vi "NI XNET CAN Signal and DAQ Logger.vi"() -> ()   [LabVIEW 2021, in "XNET-CAN-Signal-Logger.lvlib"]
uses:
  XNET-CAN-Signal-Logger.lvlib
  Typedef/Def-CAN Port Configuration.ctl
  Typedef/Def-Signal to Monitor.ctl
  Typedef/Def-DAQ AI Configuration.ctl
  Typedef/Def-Logging State.ctl
  Typedef/Def-Data Queue Ref.ctl
  Typedef/Def-Data Queue Type.ctl
  <userlib>/_NEVSTOP/NEVSTOP_TimerEngine/_Typedef/Timer-UserEvent.ctl
  Typedef/Def-GSTOP.ctl
  SubVIs/Global Variables.vi
  <userlib>/_NEVSTOP/GlobalStop/_gStop.vi
  <resource>/objmgr/xnet.rc
  <userlib>/_NEVSTOP/GlobalStop/GSTOP.lvlib
  <userlib>/_NEVSTOP/NEVSTOP_TimerEngine/TimerEngine.lvclass
panel:
  out "File size":i64 caption="File size:" format="%.0f MB"
  out "State":string caption="State:"
  in  "Tab Control":enum32{"CAN", "Analog Input"}(tab)
  in  "CAN Configurations":T1[](array[typedef]) {"Sample Rate (Hz)" format="%#_13g"}
  in  "DAQ AI Configurations":T2[](array[typedef]) {"Terminal Config" items=["Default"=-1, "RSE"=10083, "NRSE"=10078, "Differential"=10106, "Pseudodifferential"=12529]; "Min (V)" format="%#_13g"; "Max (V)" format="%#_13g"; "Sample Rate (Hz)" format="%#_13g"}
  in  "Stop Logging":bool
  in  "Signal to Monitor":T3[](array[typedef])
  out "# elements in queue":i32 caption="# elements in queue:"
  in  "Start Logging":bool
  out "Preview":string caption="Preview:"
  in  "Log file name":string="LogFile_{Year}-{Month}-{Day}-{Hour}-{Minute}-{Second}.tdms"
  in  "Log file folder":path=path "C:/Users/NI/Desktop/Data"
  in  "Exit":bool
  in  "Segment Files":bool=TRUE
  in  "Segment File Size":i64=100 caption="Seg File Size" format="%.0f MB"
  # "Configuration"
  # "Signals to Monitor"
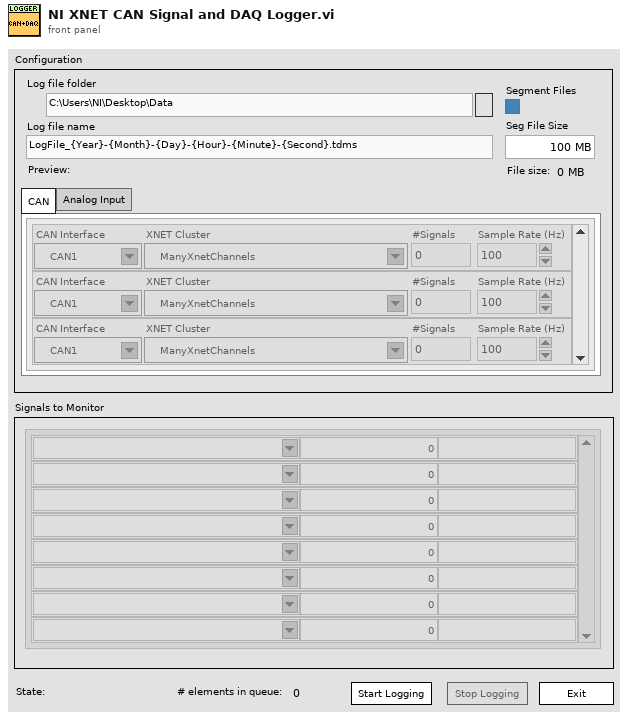
[diagram p1: front panel]
types:
  T1 = typedef "XNET-CAN-Signal-Logger.lvlib/Def-CAN Port Configuration.ctl" = cluster{"CAN Interface":refnum<k21>, "XNET Cluster":refnum<k21>, "#Signals":i32, "Sample Rate (Hz)":dbl}
  T2 = typedef "XNET-CAN-Signal-Logger.lvlib/Def-DAQ AI Configuration.ctl" = cluster{"AI Channels":tag, "Min (V)":dbl, "Max (V)":dbl, "Terminal Config":i32, "Sample Rate (Hz)":dbl, "#Samples":i32}
  T3 = typedef "XNET-CAN-Signal-Logger.lvlib/Def-Signal to Monitor.ctl" = cluster{"Name":string, "Value":dbl, "Unit":string}
  T4 = enum32{"Invalid", "Standard", "Closed", "Hidden", "Minimized", "Maximized"}
  T5 = enum32{"invalid app kind", "Development System", "Run Time System", "Student Edition", "Embedded LabVIEW", "Evaluation", "Custom"}
  T6 = enum8{"Enabled", "Disabled", "Disabled and Grayed Out"}
  T7 = typedef "XNET-CAN-Signal-Logger.lvlib/Def-Logging State.ctl" = enum16{"Configuring", "Logging..."}
  T8 = typedef "XNET-CAN-Signal-Logger.lvlib/Def-Data Queue Type.ctl" = cluster{"PackageID":i32, "Data":waveform(dbl)[]}
  T9 = typedef "XNET-CAN-Signal-Logger.lvlib/Def-GSTOP.ctl" = enum16{"Writer", "Readers"}
  T10 = typedef "XNET-CAN-Signal-Logger.lvlib/Def-Data Queue Ref.ctl" = refnum<queue>
  T11 = cluster{"Core":cluster{"Current VI Reference":refnum<vi>, "Close Panel on Exit?":bool}, "Logging State":T7, "LogFilePath":path, "Data Queue Ref":T10, "Error Queue Ref":refnum<queue>, "Monitor.SignalNames":string[], "Monitor.SignalUnits":string[]}
  T12 = cluster{"Current VI Reference":refnum<vi>, "Close Panel on Exit?":bool}
  T13 = typedef "TimerEngine.lvlib/TimerEngine.lvclass/Timer-UserEvent.ctl" = refnum<user-event>
  T14 = typedef "TimerEngine.lvlib/TimerEngine.lvclass/Timer-Userevent.ctl" = refnum<user-event>
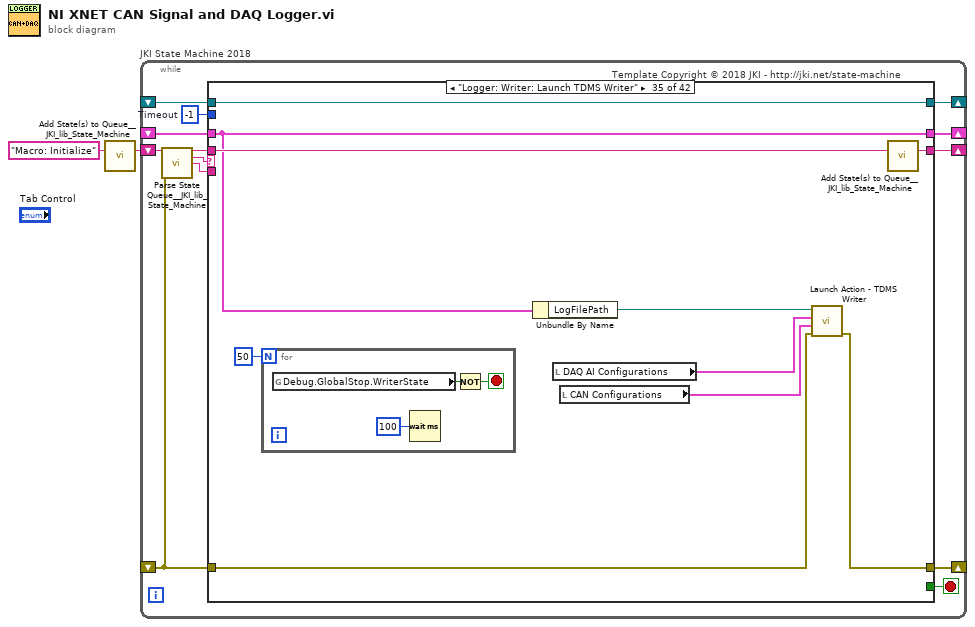
[diagram p0: block diagram]
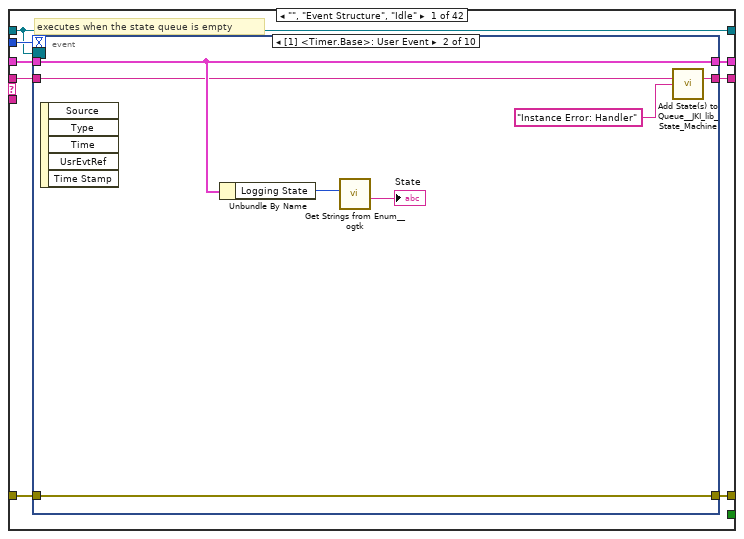
[diagram p2: hidden frame]
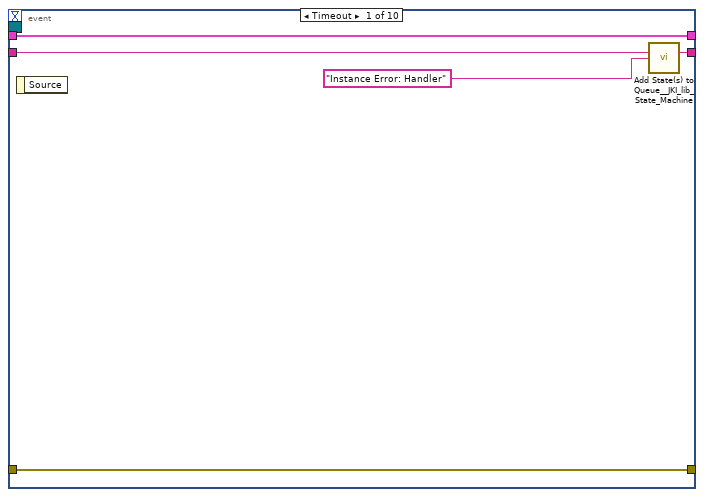
[diagram p3: hidden frame]
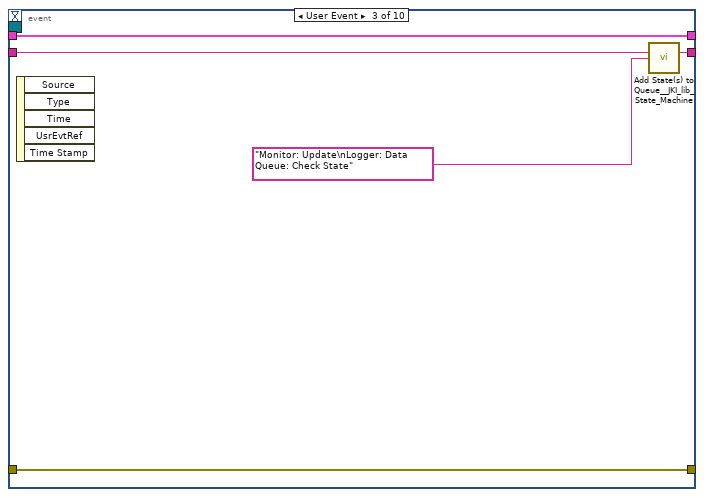
[diagram p4: hidden frame]
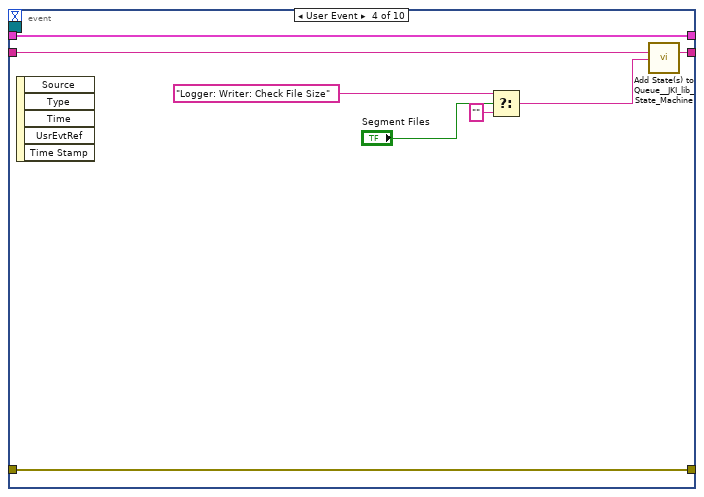
[diagram p5: hidden frame]
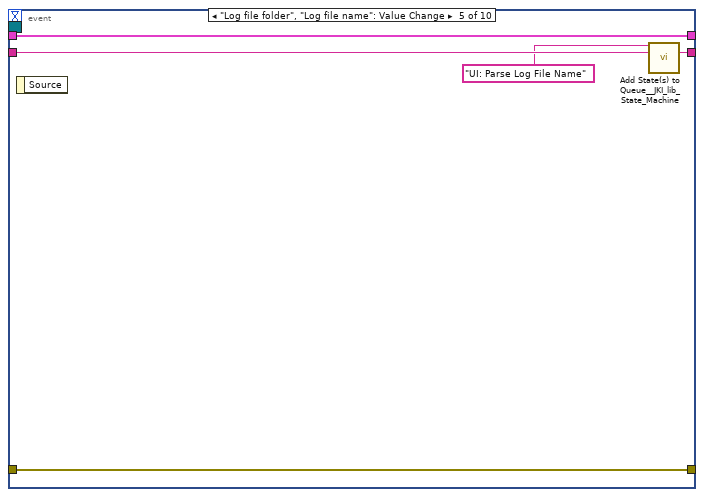
[diagram p6: hidden frame]
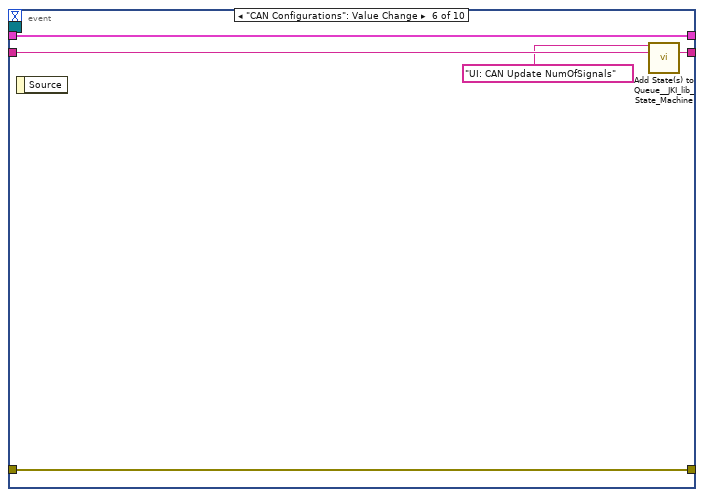
[diagram p7: hidden frame]
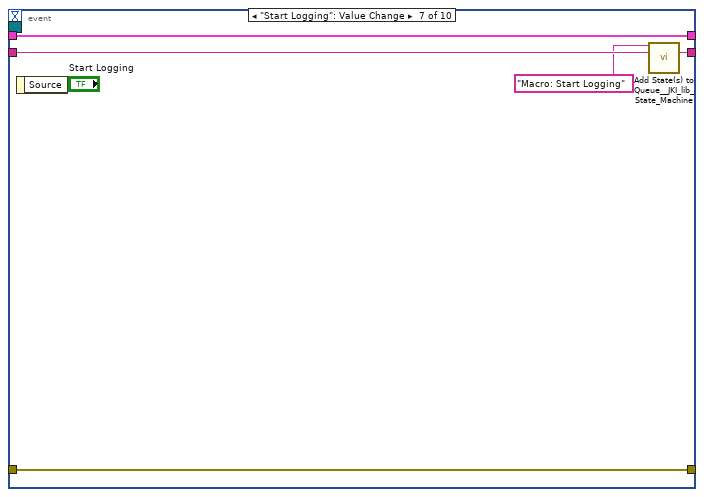
[diagram p8: hidden frame]
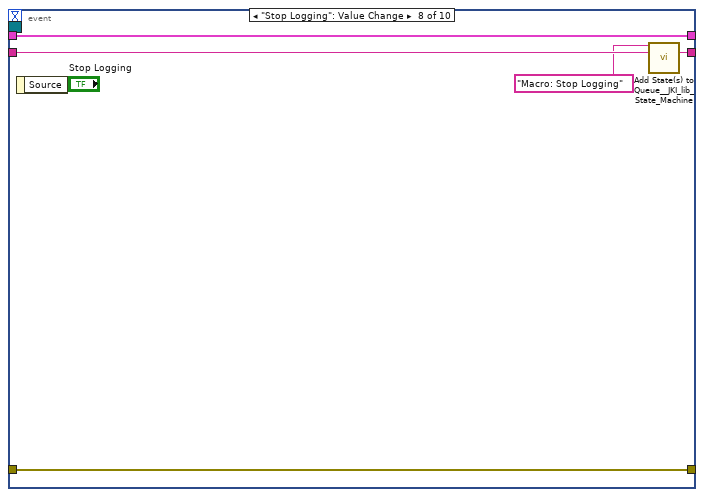
[diagram p9: hidden frame]
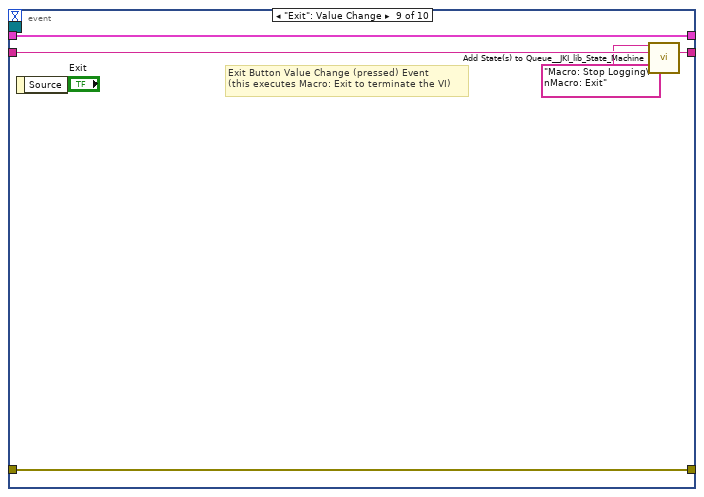
[diagram p10: hidden frame]
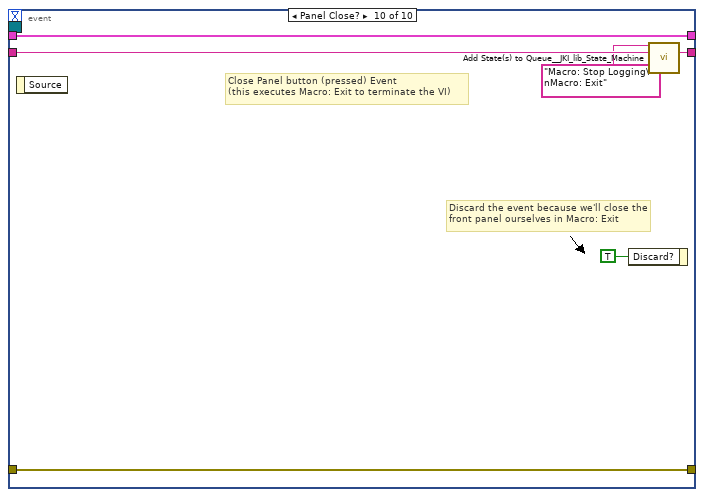
[diagram p11: hidden frame]
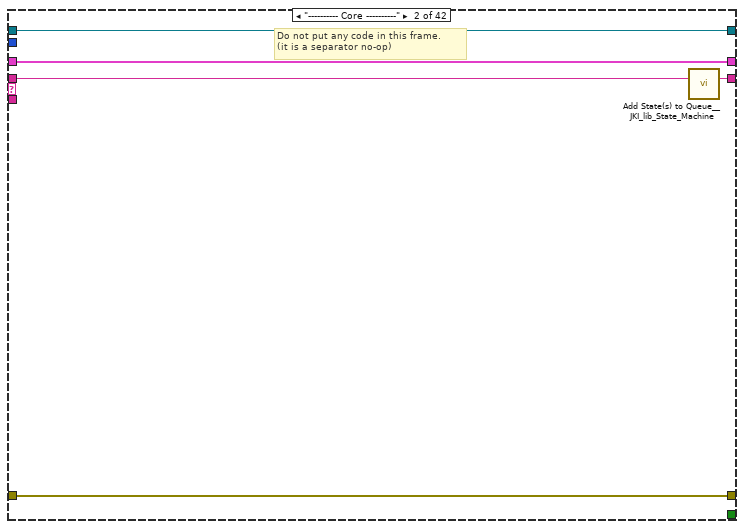
[diagram p12: hidden frame]
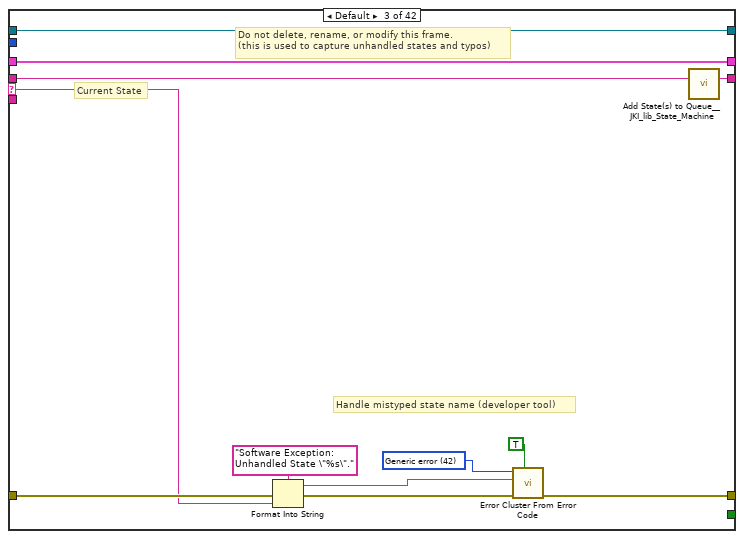
[diagram p13: hidden frame]
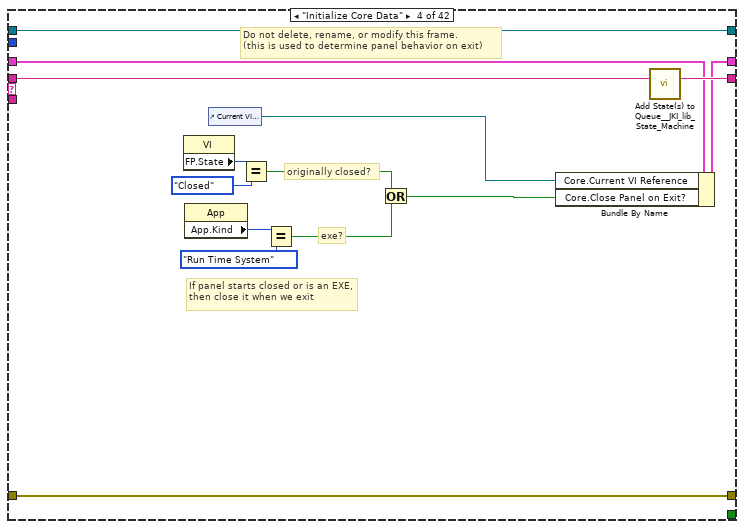
[diagram p14: hidden frame]
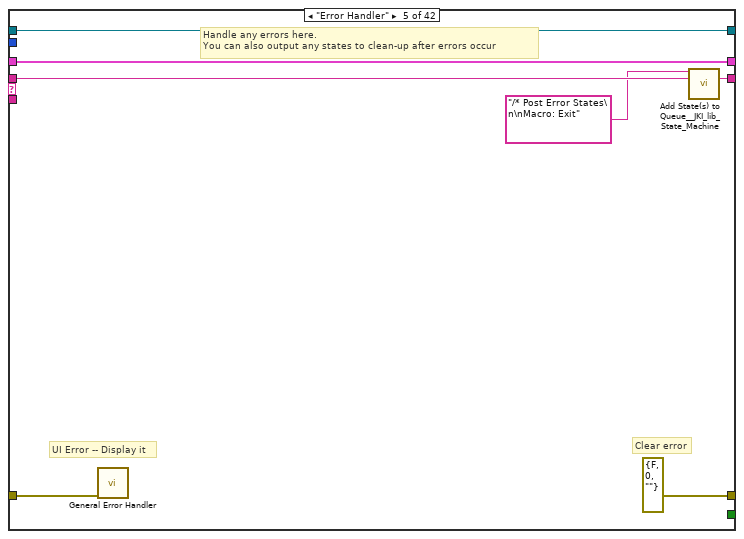
[diagram p15: hidden frame]
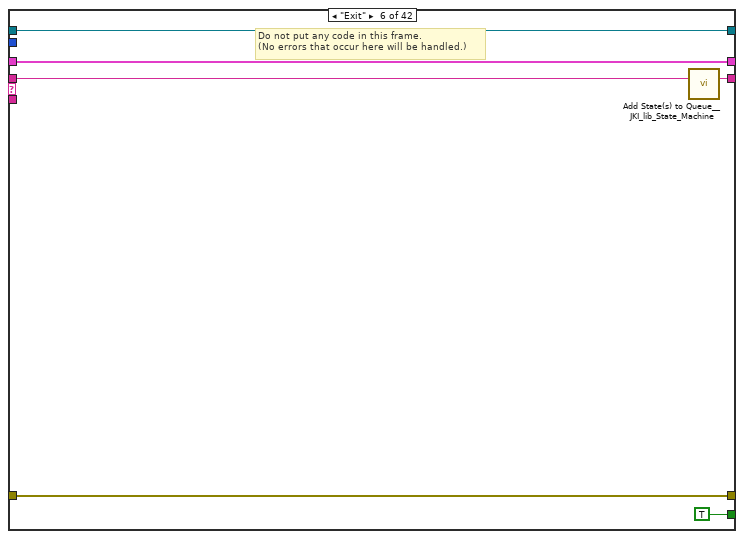
[diagram p16: hidden frame]
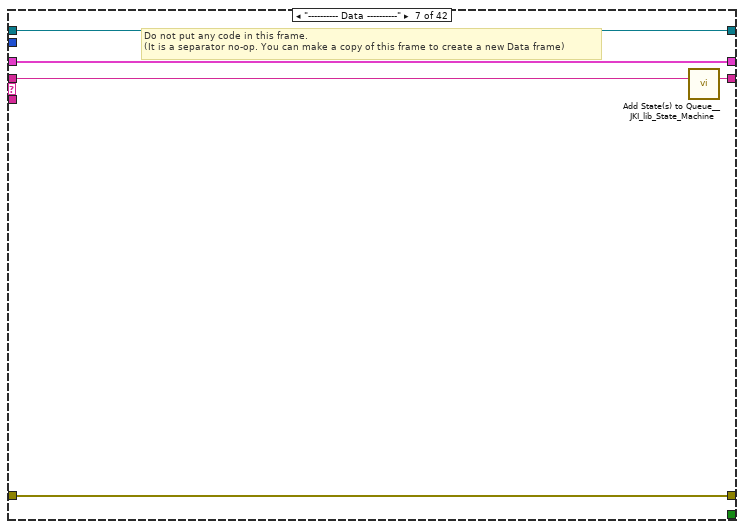
[diagram p17: hidden frame]
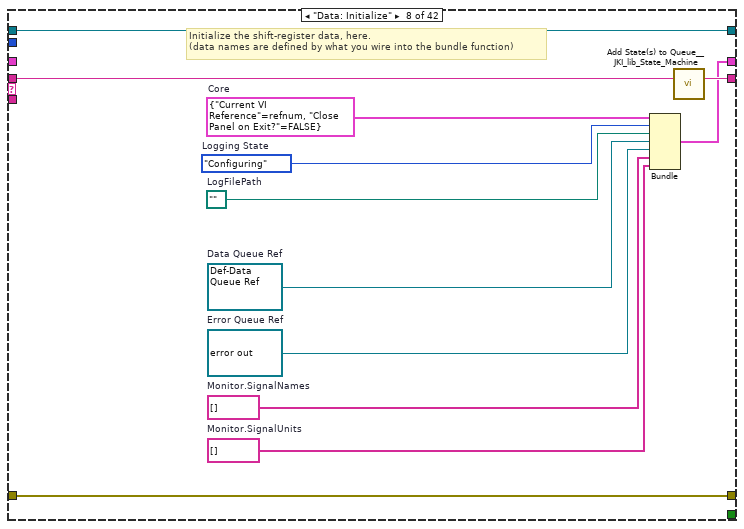
[diagram p18: hidden frame]
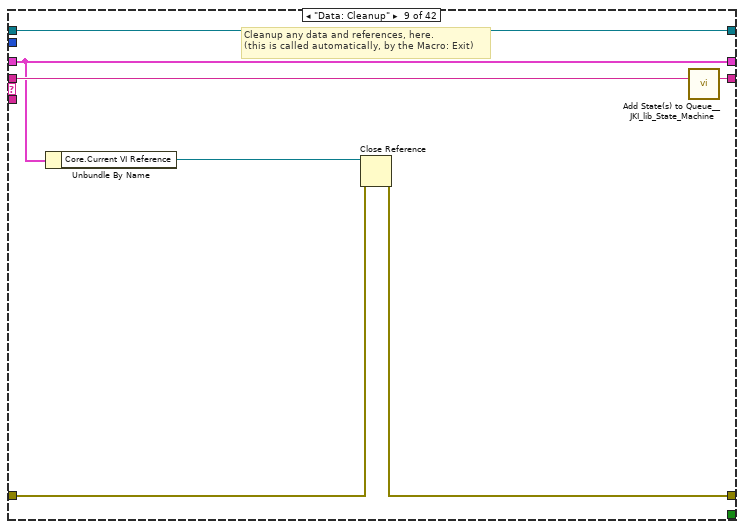
[diagram p19: hidden frame]
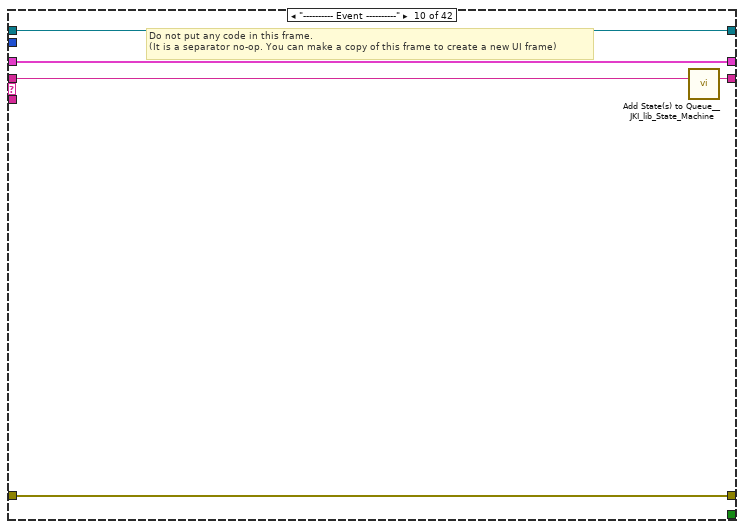
[diagram p20: hidden frame]
diagram:
  n1 = call <vilib>:"Add State(s) to Queue__JKI_lib_State_Machine.vi"("State(s) in (\"\")"="Macro: Initialize") -> ("States Out"=w2:string)  [unwired: 14 in]
  n2 = while "JKI State Machine 2018" {
    shift-right: [w8] -> _
    shift-left: _ -> [w7]
    shift-right: [w11] -> _
    shift-left: _ -> [w5]
    shift-right: [w10] -> _
    shift-left: w2 -> [w12]
    shift-right: [w4] -> _
    shift-left: _ -> [w3]
    stop <- w9 stop-if-true
    w6 = -1  # Timeout
    # "Template Copyright © 2018 JKI - http://jki.net/state-machine"
    n3 = call <vilib>:"Parse State Queue__JKI_lib_State_Machine.vi"("State Queue"=w12, "Error In (no error)"=w5) -> ("Remaining States"=w14:string, "Current State"=w15:string, "Arguments"=w13:string)  [unwired: 11 in]
    n4 = case shown="\"Logger: Writer: Launch TDMS Writer\"" w15 {
      selector: w15 -> [_ _ w86 _ _ _ _ _ _ _ _ _ _ _ _ _ _ _ _ _ _ _ _ _ _ _ _ _ _ _ _ _ _ _ _ _ _ _ _ _ _ _]
      tunnel: w14 -> [w23 w84 w90 w110 w117 w123 w128 w140 w147 w152 w180 w189 w203 w209 w217 w224 w236 w310 w327 w334 w344 w350 w358 w366 w372 w383 w388 w397 w404 w413 w418 w428 w435 w443 w453 w472 w480 w489 w496 w511 w531 w542]
      tunnel: w13 -> [_ _ _ _ _ _ _ _ _ _ _ _ w194 _ _ w219 w230 _ _ _ _ _ _ _ _ _ _ _ _ _ _ _ _ _ _ _ _ _ w493 _ _ _]
      tunnel: w7 -> [w21 w81 w88 w103 w114 w121 w125 _ w142 w149 w178 w187 w201 w206 w215 w222 w232 w307 w324 w331 w341 w347 w355 w363 w369 w380 w385 w395 w402 w411 w415 w426 w433 w441 w451 w470 w478 w487 w494 w508 w528 w538]
      tunnel: [w20 w82 w92 w107 errorcluster {"status"=FALSE, "code"=0, "source"=""} ("error out") w120 w126 w137 w143 w150 w176 w181 w195 w207 w214 w220 w233 w308 w325 w332 w342 w348 w356 w364 w370 w381 w386 w393 w399 w407 w416 w422 w430 w438 w448 w458 w476 w485 w491 w509 w521 w539] -> w11
      tunnel: w5 -> [w19 w82 w91 w107 w113 w120 w126 w137 w144 w150 w166 w185 w197 w207 w214 w221 w234 w308 w325 w332 w342 w348 w356 w364 w370 w381 w386 w391 w400 w409 w416 w423 w431 w439 w449 w468 w477 w486 w492 w509 w526 w540]
      tunnel: [w22 w83 w89 w109 w116 w122 w127 w139 w146 w151 w179 w188 w202 w208 w216 w223 w235 w309 w326 w333 w343 w349 w357 w365 w371 w382 w387 w396 w403 w412 w417 w427 w434 w442 w452 w471 w479 w488 w495 w510 w530 w541] -> w10
      tunnel: [_ _ _ _ _ TRUE _ _ _ _ _ _ _ _ _ _ _ _ _ _ _ _ _ _ _ _ _ _ _ _ _ _ _ _ _ _ _ _ _ _ _ _] -> w9
      tunnel: [w18 w81 w88 w108 w114 w121 w125 w138 w142 w149 w178 w187 w201 w206 w215 w222 w232 w307 w320 w331 w341 w347 w353 w361 w369 w380 w385 w392 w402 w411 w415 w421 w433 w441 w451 w470 w478 w487 w494 w508 w527 w538] -> w8
      tunnel: w6 -> [w17 _ _ _ _ _ _ _ _ _ _ _ _ _ _ _ _ _ _ _ _ _ _ _ _ _ _ _ _ _ _ _ _ _ _ _ _ _ _ _ _ _]
      tunnel: [w16 w80 w85 w97 w111 w118 w124 w129 w141 w148 w177 w186 w196 w205 w211 w218 w229 w303 w318 w328 w340 w345 w351 w359 w367 w373 w384 w389 w398 w405 w414 w419 w429 w436 w445 w464 w473 w481 w490 w507 w515 w532] -> w4
      tunnel: w3 -> [w16 w80 w85 w97 w111 w118 w124 w129 w141 w148 _ w186 w196 w205 w211 w218 w229 w303 w318 w328 w340 w345 w351 w359 w367 w373 w384 w389 w398 w405 w414 w419 w429 w436 w445 w464 w473 w481 w490 w507 w515 w532]
      frame "", "Event Structure", "Idle" {
        # "executes when the state queue is empty"
        n5 = event shown="[1] <Timer.Base>: User Event" {
          selector: w16 -> [_ _ _ _ _ _ _ _ _ _]
          dyn-events: _ -> [_ _ _ _ _ _ _ _ _ _]
          timeout: w17 -> [_ _ _ _ _ _ _ _ _ _]
          tunnel: w23 -> [w25 w32 w36 w41 w53 w58 w63 w68 w73 w79]
          tunnel: [w28 w35 w40 w48 w52 w57 w62 w67 w72 w78] -> w22
          tunnel: w21 -> [w26 w33 w38 w46 w50 w55 w59 w64 w70 w76]
          tunnel: [w27 w34 w39 w47 w51 w56 w61 w66 w71 w77] -> w20
          tunnel: w19 -> [w27 w34 w39 w47 w51 w56 w61 w66 w71 w77]
          tunnel: [w26 w33 w38 w46 w50 w55 w59 w64 w70 w76] -> w18
          event Timeout {
            n6 = event-data() -> ()  [unwired: 1 in, 1 out]
            n7 = call <vilib>:"Add State(s) to Queue__JKI_lib_State_Machine.vi"("State(s) in (\"\")"=w25, "State(s) at Back (\"\")"="Instance Error: Handler" ("string")) -> ("States Out"=w28:string)  [unwired: 13 in]
          }
          event User Event {
            n8 = event-data() -> ()  [unwired: 1 in, 5 out]
            n9 = Unbundle By Name(w33) -> ("Logging State"=w30:T7)
            n10 = call <userlib>:"Get Strings from Enum__ogtk.vi"("Enum"=w30) -> ("String Value"=→"State":string)  [unwired: 7 in, 3 out]
            n11 = call <vilib>:"Add State(s) to Queue__JKI_lib_State_Machine.vi"("State(s) in (\"\")"=w32, "State(s) at Back (\"\")"="Instance Error: Handler" ("string")) -> ("States Out"=w35:string)  [unwired: 13 in]
          }
          event User Event {
            n12 = event-data() -> ()  [unwired: 1 in, 5 out]
            n13 = call <vilib>:"Add State(s) to Queue__JKI_lib_State_Machine.vi"("State(s) in (\"\")"=w36, "State(s) at Back (\"\")"="Monitor: Update\nLogger: Data Queue: Check State" ("State(s) at Back (\"\")")) -> ("States Out"=w40:string)  [unwired: 13 in]
          }
          event User Event {
            n14 = event-data() -> ()  [unwired: 1 in, 5 out]
            n15 = Select(t="Logger: Writer: Check File Size" ("State(s) at Back (\"\")"), s="Segment Files", f="") -> (s? t:f=w44:string)
            n16 = call <vilib>:"Add State(s) to Queue__JKI_lib_State_Machine.vi"("State(s) in (\"\")"=w41, "State(s) at Back (\"\")"=w44) -> ("States Out"=w48:string)  [unwired: 13 in]
          }
          event "Log file folder", "Log file name": Value Change {
            n17 = event-data() -> ()  [unwired: 1 in, 1 out]
            n18 = call <vilib>:"Add State(s) to Queue__JKI_lib_State_Machine.vi"("State(s) in Front (\"\")"="UI: Parse Log File Name", "State(s) in (\"\")"=w53) -> ("States Out"=w52:string)  [unwired: 13 in]
          }
          event "CAN Configurations": Value Change {
            n19 = event-data() -> ()  [unwired: 1 in, 1 out]
            n20 = call <vilib>:"Add State(s) to Queue__JKI_lib_State_Machine.vi"("State(s) in Front (\"\")"="UI: CAN Update NumOfSignals", "State(s) in (\"\")"=w58) -> ("States Out"=w57:string)  [unwired: 13 in]
          }
          event "Start Logging": Value Change {
            n21 = event-data() -> ()  [unwired: 1 in, 1 out]
            n22 = call <vilib>:"Add State(s) to Queue__JKI_lib_State_Machine.vi"("State(s) in Front (\"\")"="Macro: Start Logging", "State(s) in (\"\")"=w63) -> ("States Out"=w62:string)  [unwired: 13 in]
          }
          event "Stop Logging": Value Change {
            n23 = event-data() -> ()  [unwired: 1 in, 1 out]
            n24 = call <vilib>:"Add State(s) to Queue__JKI_lib_State_Machine.vi"("State(s) in Front (\"\")"="Macro: Stop Logging", "State(s) in (\"\")"=w68) -> ("States Out"=w67:string)  [unwired: 13 in]
          }
          event "Exit": Value Change {
            # "Exit Button Value Change (pressed) Event\n(this executes Macro: Exit to terminate the VI)"
            n25 = event-data() -> ()  [unwired: 1 in, 1 out]
            n26 = call <vilib>:"Add State(s) to Queue__JKI_lib_State_Machine.vi"("State(s) in Front (\"\")"="Macro: Stop Logging\nMacro: Exit", "State(s) in (\"\")"=w73) -> ("States Out"=w72:string)  [unwired: 13 in]
          }
          event Panel Close? {
            # "Discard the event because we'll close the front panel ourselves in Macro: Exit"
            # "Close Panel button (pressed) Event\n(this executes Macro: Exit to terminate the VI)"
            n27 = event-data() -> ()  [unwired: 1 in, 1 out]
            n28 = event-data("Discard?"=TRUE) -> ()  [unwired: 1 in, 1 out]
            n29 = call <vilib>:"Add State(s) to Queue__JKI_lib_State_Machine.vi"("State(s) in Front (\"\")"="Macro: Stop Logging\nMacro: Exit", "State(s) in (\"\")"=w79) -> ("States Out"=w78:string)  [unwired: 13 in]
          }
        }
      }
      frame "---------- Core ----------" {
        # "Do not put any code in this frame.\n(it is a separator no-op)"
        n30 = call <vilib>:"Add State(s) to Queue__JKI_lib_State_Machine.vi"("State(s) in (\"\")"=w84) -> ("States Out"=w83:string)  [unwired: 14 in]
      }
      frame Default {
        w95 = 42 items=["No error", "Argument error", "Memory is full", "Out of zone", "End of file", "File already open", "Generic file I/O error", "File not found", "File permission error", "Disk is full", "Duplicate path", "Too many files open", "System feature not enabled", "Resource file not found", "Cannot add resource", "Resource not found", "Image not found", "Image memory error", "Pen does not exist", "Config type invalid", "Config token not found", "Config parse error", "Config memory error", "Bad external code format", "Bad external code offset", "External code not present", "Null window", "Destroy window error", "Null menu", "Print aborted", "Bad print record", "Print driver error", "Windows error during printing", "Memory error during printing", "Print dialog error", "Generic print error", "Invalid device refnum", "Device not found", "Device parameter error", "Device unit error", "Cannot open device", "Device call aborted", "Generic error", "Cancelled by user", "Object ID too low", "Object ID too high", "Object not in heap", "Unknown heap", "Unknown object (invalid DefProc)", "Unknown object (DefProc not in table)", "Message out of range", "Invalid (null) method", "Unknown message", "Manager call not supported", "Bad address", "Network operation in progress", "Network operation timed out", "Connection is busy", "Network attribute not supported", "Network error", "Address in use", "System out of memory", "Connection aborted", "Connection refused", "Not connected", "Already connected", "Connection closed", "Initialization error (interapplication manager)", "Bad occurrence", "Wait on unbound occurrence handler", "Occurrence queue overflow", "Datalog type conflict", "Unused", "Unrecognized type (interapplication manager)", "Memory corrupt", "Failed to make temporary DLL", "Old CIN version", "Drag socket not found", "Failed to load drop-object", "Failed to register OLE object", "Failed to release OLE object", "Format specifier type mismatch", "Unknown format specifier", "Too few format specifiers", "Too many format specifiers", "Scan failed", "Newer CIN version", "Error converting to variant", "Runtime menu error", "Password tampered", "Variant attribute not found", "Incompatible variant data type", "Event data is not available", "Event Store is not present", "Occurrence is not found", "Event Queue is not created", "Event info is not available", "Refnum passed is NULL", "Error retrieving Class GUID", "Error retrieving CoClass GUID", "Error retrieving TypeLib GUID.", "Bad built application magic bytes.", "Specific driver is different from the specific driver associated with the Logical Name.", "There is no session opened to the class driver.", "Max Error", "MAX - Error with config objects", "MAX - Error loading configuration", "MAX - Group not supported"]
        # "Current State"
        # "Do not delete, rename, or modify this frame.\n(this is used to capture unhandled states and typos)"
        # "Handle mistyped state name (developer tool)"
        n31 = Format Into String(format string="Software Exception: Unhandled State \"%s\"." ("message"), error in=w91, w86) -> (resulting string=w94:string, error out=w93:errorcluster)  [unwired: 1 in]
        n32 = call <vilib>:"Error Cluster From Error Code.vi"("show call chain? (False)"=TRUE, "error in (no error)"=w93, "error message (\"\")"=w94, "error code (0)"=w95) -> ("error out"=w92:errorcluster)  [unwired: 5 in]
        n33 = call <vilib>:"Add State(s) to Queue__JKI_lib_State_Machine.vi"("State(s) in (\"\")"=w90) -> ("States Out"=w89:string)  [unwired: 14 in]
      }
      frame "Initialize Core Data" {
        # "Do not delete, rename, or modify this frame.\n(this is used to determine panel behavior on exit)"
        # "originally closed?"
        # "exe?"
        # "If panel starts closed or is an EXE, then close it when we exit"
        n34 = property class="VI"() -> ("FP.State"=w100:T4)  [unwired: 2 in, 2 out]
        n35 = property class="App"() -> ("App.Kind"=w106:T5)  [unwired: 2 in, 2 out]
        n36 = control-ref of="Current VI Reference"() -> (w101:refnum<vi>)
        n37 = Equal?(x=w100, y=T4."Closed" ("Front Panel Window:State")) -> (x = y?=w98:bool)
        n38 = Equal?(x=w106, y=T5."Run Time System" ("Application:Kind")) -> (x = y?=w104:bool)
        n39 = Or(x=w98, y=w104) -> (x .or. y?=w102:bool)
        n40 = Bundle By Name(cluster=w103, "Core.Current VI Reference"=w101, "Core.Close Panel on Exit?"=w102) -> (w108:T11)
        n41 = call <vilib>:"Add State(s) to Queue__JKI_lib_State_Machine.vi"("State(s) in (\"\")"=w110) -> ("States Out"=w109:string)  [unwired: 14 in]
      }
      frame "Error Handler" {
        # "UI Error -- Display it"
        # "Handle any errors here.\nYou can also output any states to clean-up after errors occur"
        # "Clear error"
        n42 = call <vilib>:"General Error Handler.vi"("error in (no error)"=w113) -> ()  [unwired: 10 in, 5 out]
        n43 = call <vilib>:"Add State(s) to Queue__JKI_lib_State_Machine.vi"("State(s) in Front (\"\")"="/* Post Error States\n\nMacro: Exit", "State(s) in (\"\")"=w117) -> ("States Out"=w116:string)  [unwired: 13 in]
      }
      frame "Exit" {
        # "Do not put any code in this frame.\n(No errors that occur here will be handled.)"
        n44 = call <vilib>:"Add State(s) to Queue__JKI_lib_State_Machine.vi"("State(s) in (\"\")"=w123) -> ("States Out"=w122:string)  [unwired: 14 in]
      }
      frame "---------- Data ----------" {
        # "Do not put any code in this frame.\n(It is a separator no-op. You can make a copy of this frame to create a new Data frame)"
        n45 = call <vilib>:"Add State(s) to Queue__JKI_lib_State_Machine.vi"("State(s) in (\"\")"=w128) -> ("States Out"=w127:string)  [unwired: 14 in]
      }
      frame "Data: Initialize" {
        w131 = string[] []  # Monitor.SignalUnits
        w130 = string[] []  # Monitor.SignalNames
        w132 = refnum<queue> refnum  # Error Queue Ref
        w133 = T10 refnum  # Data Queue Ref
        w134 = Def-Logging_State."Configuring"  # Logging State
        w135 = path ""  # LogFilePath
        w136 = T12 {"Current VI Reference"=refnum, "Close Panel on Exit?"=FALSE}  # Core
        # "Initialize the shift-register data, here.\n(data names are defined by what you wire into the bundle function)"
        n46 = Bundle("Core"=w136, "Logging State"=w134, "LogFilePath"=w135, "Data Queue Ref"=w133, "Error Queue Ref"=w132, "Monitor.SignalNames"=w130, "Monitor.SignalUnits"=w131) -> (w138:T11)  [unwired: 1 in]
        n47 = call <vilib>:"Add State(s) to Queue__JKI_lib_State_Machine.vi"("State(s) in (\"\")"=w140) -> ("States Out"=w139:string)  [unwired: 14 in]
      }
      frame "Data: Cleanup" {
        # "Cleanup any data and references, here.\n(this is called automatically, by the Macro: Exit)"
        n48 = Unbundle By Name(w142) -> ("Core.Current VI Reference"=w145:refnum<vi>)
        n49 = Close Reference(reference=w145, error in (no error)=w144) -> (error out=w143:errorcluster)
        n50 = call <vilib>:"Add State(s) to Queue__JKI_lib_State_Machine.vi"("State(s) in (\"\")"=w147) -> ("States Out"=w146:string)  [unwired: 14 in]
      }
      frame "---------- Event ----------" {
        # "Do not put any code in this frame.\n(It is a separator no-op. You can make a copy of this frame to create a new UI frame)"
        n51 = call <vilib>:"Add State(s) to Queue__JKI_lib_State_Machine.vi"("State(s) in (\"\")"=w152) -> ("States Out"=w151:string)  [unwired: 14 in]
      }
      frame "Event: Register" {
        w157 = T13 refnum  # Timer.TDMSFileSegment
        w160 = T13 refnum  # Timer.Monitor
        w161 = T13 refnum  # Timer.Base
        w169 = FALSE ("Start Imidiatlely?(T)")
        # "Do not put any code in this frame.\n(It is a separator no-op. You can make a copy of this frame to create a new UI frame)"
        n52 = global read "Global Variables.vi" "Const.Timer.TDMSFileSegment"() -> (w173:string)
        n53 = global read "Global Variables.vi" "Const.Timer.Base"() -> (w167:string)
        n54 = global read "Global Variables.vi" "Const.Timer.Monitor"() -> (w175:string)
        n55 = call <userlib>:"Register.vi"("error in (no error)"=w166, "TimePeroid(ms)"=200, "Name"=w167) -> ("error out"=w165:errorcluster, "TimeupEvent"=w163:T14)  [unwired: 7 in]
        n56 = To Variant(anything=w163) -> (Variant=w164:variant)
        n57 = Variant To Data(type=w161, Variant=w164) -> (data=w162:T13)  [unwired: 1 in, 1 out]
        n58 = call <userlib>:"Register.vi"("Start Imidiatlely?(T)"=w169, "error in (no error)"=w165, "TimePeroid(ms)"=200, "Name"=w175) -> ("error out"=w174:errorcluster, "TimeupEvent"=w154:T14)  [unwired: 6 in]
        n59 = To Variant(anything=w154) -> (Variant=w159:variant)
        n60 = Variant To Data(type=w160, Variant=w159) -> (data=w153:T13)  [unwired: 1 in, 1 out]
        n61 = call <userlib>:"Register.vi"("Start Imidiatlely?(T)"=w169, "error in (no error)"=w174, "TimePeroid(ms)"=1000, "Name"=w173) -> ("error out"=w170:errorcluster, "TimeupEvent"=w156:T14)  [unwired: 6 in]
        n62 = To Variant(anything=w156) -> (Variant=w158:variant)
        n63 = Variant To Data(type=w157, Variant=w158) -> (data=w155:T13)  [unwired: 1 in, 1 out]
        n64 = register-events(error in=w170, w162, w153, w155) -> (reference out=w177:refnum<event-registration>, error out=w176:errorcluster)  [unwired: 1 in]
        n65 = call <vilib>:"Add State(s) to Queue__JKI_lib_State_Machine.vi"("State(s) in (\"\")"=w180) -> ("States Out"=w179:string)  [unwired: 14 in]
      }
      frame "Event: Unregister" {
        # "Do not put any code in this frame.\n(It is a separator no-op. You can make a copy of this frame to create a new UI frame)"
        n66 = Unregister For Events(event registration refnum=w186, error in=w185) -> (error out=w182:errorcluster)
        n67 = call <userlib>:"List Timers.vi"("error in (no error)"=w182) -> ("error out"=w184:errorcluster, "Timers"=w183:string[])  [unwired: 8 in, 1 out]
        n68 = for {
          tunnel: w183 -> [w191] mode=indexing
          shift-right: [w190] -> w181
          shift-left: w184 -> [w192]
          n69 = call <userlib>:"Unregister.vi"("error in (no error)"=w192, "Name"=w191) -> ("error out"=w190:errorcluster)  [unwired: 9 in]
        }
        n70 = call <vilib>:"Add State(s) to Queue__JKI_lib_State_Machine.vi"("State(s) in (\"\")"=w189) -> ("States Out"=w188:string)  [unwired: 14 in]
      }
      frame "Event: Control Timers" {
        n71 = case shown="\"Start\"" w194 {
          tunnel: [_ TRUE ("Start Imidiatlely?(T)")] -> w193
          frame "Stop", Default {
          }
          frame "Start" {
          }
        }
        n72 = global read "Global Variables.vi" "Const.Timer.TDMSFileSegment"() -> (w198:string)
        n73 = global read "Global Variables.vi" "Const.Timer.Monitor"() -> (w200:string)
        n74 = call <userlib>:"Enable.vi"("error in (no error)"=w197, "Enable?"=w193, "Name"=w200) -> ("error out"=w199:errorcluster)  [unwired: 8 in]
        n75 = call <userlib>:"Enable.vi"("error in (no error)"=w199, "Enable?"=w193, "Name"=w198) -> ("error out"=w195:errorcluster)  [unwired: 8 in]
        n76 = call <vilib>:"Add State(s) to Queue__JKI_lib_State_Machine.vi"("State(s) in (\"\")"=w203) -> ("States Out"=w202:string)  [unwired: 14 in]
      }
      frame "---------- UI ----------" {
        # "Do not put any code in this frame.\n(It is a separator no-op. You can make a copy of this frame to create a new UI frame)"
        n77 = call <vilib>:"Add State(s) to Queue__JKI_lib_State_Machine.vi"("State(s) in (\"\")"=w209) -> ("States Out"=w208:string)  [unwired: 14 in]
      }
      frame "UI: Initialize" {
        # "Initialize the User Interface, here.\n(this is called automatically, by the Macro: Init)"
        n78 = local write "# elements in queue"(0 ("# elements in queue:")) -> ()
        n79 = local write "File size"(i64 0 ("File size")) -> ()
        n80 = call <vilib>:"Add State(s) to Queue__JKI_lib_State_Machine.vi"("State(s) in Front (\"\")"="UI: Toggle Logging State\nUI: Parse Log File Name\nUI: CAN Update NumOfSignals" ("State(s) in Front (\"\")"), "State(s) in (\"\")"=w217) -> ("States Out"=w216:string)  [unwired: 13 in]
      }
      frame "UI: Cursor Set" {
        # "Argument"
        # "Set and Unset Cursor Busy.\n(Usage: \"UI: Cursor Set >> Busy|Idle\")"
        n81 = case shown="\"Idle\", Default" w219 {
          tunnel: w221 -> [w226 w228]
          tunnel: [w225 w227] -> w220
          frame "Idle", Default {
            n82 = call <vilib>:"Unset Busy.vi"("error in (no error)"=w226) -> ("error out"=w225:errorcluster)  [unwired: 10 in]
          }
          frame "Busy" {
            n83 = call <vilib>:"Set Busy.vi"("error in (no error)"=w228) -> ("error out"=w227:errorcluster)  [unwired: 9 in, 1 out]
          }
        }
        n84 = call <vilib>:"Add State(s) to Queue__JKI_lib_State_Machine.vi"("State(s) in (\"\")"=w224) -> ("States Out"=w223:string)  [unwired: 14 in]
      }
      frame "UI: Front Panel State" {
        # "Argument"
        # "Set Front Panel Open or Closed\n(Usage: \"UI: Front Panel State >> Open|Close\")"
        n85 = Unbundle By Name(w232) -> ("Core.Current VI Reference"=w231:refnum<vi>)
        n86 = case shown="\"Minimize\", \"Minimized\"" w230 {
          tunnel: w234 -> [w242 w257 w268 w281 w294]
          tunnel: [w244 w258 w270 w283 w296] -> w233
          tunnel: w231 -> [w243 w255 w269 w282 w295]
          frame "Open", "Standard", Default {
            w237 = T4."Standard" ("State")
            n87 = property class="VI"(reference=w243, error in=w242) -> (reference out=w240:refnum<vi>, error out=w241:errorcluster, "FP.State"=w239:T4)
            n88 = Not Equal?(x=w239, y=w237) -> (x != y?=w238:bool)
            n89 = case shown="True" w238 {
              tunnel: [w248 w250] -> w244
              tunnel: w241 -> [w247 w250]
              tunnel: w240 -> [w246 _]
              tunnel: w237 -> [w245 _]
              frame True {
                n90 = invoke class="VI" method="FP.Open"(reference=w246, error in=w247, "Activate"=TRUE, "State"=w245) -> (error out=w248:errorcluster)  [unwired: 1 in, 4 out]
              }
              frame False {
              }
            }
          }
          frame "Close", "Closed" {
            n91 = property class="VI"(reference=w255, error in=w257) -> (reference out=w254:refnum<vi>, error out=w256:errorcluster, "FP.State"=w252:T4)
            n92 = Not Equal?(x=w252, y=T4."Closed" ("Front Panel Window:State")) -> (x != y?=w251:bool)
            n93 = case shown="True" w251 {
              tunnel: [w259 w262] -> w258
              tunnel: w256 -> [w259 w261]
              tunnel: w254 -> [_ w260]
              frame False {
              }
              frame True {
                n94 = invoke class="VI" method="FP.Close"(reference=w260, error in=w261) -> (error out=w262:errorcluster)  [unwired: 1 in, 2 out]
              }
            }
          }
          frame "Hidden", "Hide" {
            w263 = T4."Hidden" ("State")
            n95 = property class="VI"(reference=w269, error in=w268) -> (reference out=w266:refnum<vi>, error out=w267:errorcluster, "FP.State"=w265:T4)
            n96 = Not Equal?(x=w265, y=w263) -> (x != y?=w264:bool)
            n97 = case shown="True" w264 {
              tunnel: [w274 w275] -> w270
              tunnel: w267 -> [w273 w275]
              tunnel: w266 -> [w272 _]
              tunnel: w263 -> [w271 _]
              frame True {
                n98 = invoke class="VI" method="FP.Open"(reference=w272, error in=w273, "State"=w271) -> (error out=w274:errorcluster)  [unwired: 2 in, 4 out]
              }
              frame False {
              }
            }
          }
          frame "Minimize", "Minimized" {
            w276 = T4."Minimized" ("State")
            n99 = property class="VI"(reference=w282, error in=w281) -> (reference out=w279:refnum<vi>, error out=w280:errorcluster, "FP.State"=w278:T4)
            n100 = Not Equal?(x=w278, y=w276) -> (x != y?=w277:bool)
            n101 = case shown="True" w277 {
              tunnel: [w287 w288] -> w283
              tunnel: w280 -> [w286 w288]
              tunnel: w279 -> [w285 _]
              tunnel: w276 -> [w284 _]
              frame True {
                n102 = invoke class="VI" method="FP.Open"(reference=w285, error in=w286, "State"=w284) -> (error out=w287:errorcluster)  [unwired: 2 in, 4 out]
              }
              frame False {
              }
            }
          }
          frame "Maximize", "Maximized" {
            w289 = T4."Maximized" ("State")
            n103 = property class="VI"(reference=w295, error in=w294) -> (reference out=w292:refnum<vi>, error out=w293:errorcluster, "FP.State"=w291:T4)
            n104 = Not Equal?(x=w291, y=w289) -> (x != y?=w290:bool)
            n105 = case shown="True" w290 {
              tunnel: [w300 w301] -> w296
              tunnel: w293 -> [w299 w301]
              tunnel: w292 -> [w298 _]
              tunnel: w289 -> [w297 _]
              frame True {
                n106 = invoke class="VI" method="FP.Open"(reference=w298, error in=w299, "State"=w297) -> (error out=w300:errorcluster)  [unwired: 2 in, 4 out]
              }
              frame False {
              }
            }
          }
        }
        n107 = call <vilib>:"Add State(s) to Queue__JKI_lib_State_Machine.vi"("State(s) in (\"\")"=w236) -> ("States Out"=w235:string)  [unwired: 14 in]
      }
      frame "UI: Toggle Logging State" {
        n108 = Unbundle By Name(w307) -> ("Logging State"=w306:T7)
        n109 = case shown="\"Configuring\"" w306 {
          tunnel: [w313 T6."Disabled and Grayed Out" ("Disabled")] -> w302
          tunnel: [T6."Disabled and Grayed Out" ("Disabled") T6."Enabled" ("Disabled")] -> w305
          tunnel: [w313 T6."Disabled" ("Disabled")] -> w304
          frame "Configuring" {
            w313 = T6."Enabled" ("Disabled")
          }
          frame "Logging..." {
          }
        }
        n110 = property on="Log file folder" class="Path"("DisabledEnum"=w302) -> ()  [unwired: 2 in, 2 out]
        n111 = property on="Log file name" class="Str"("DisabledEnum"=w302) -> ()  [unwired: 2 in, 2 out]
        n112 = property on="Segment Files" class="Bool (strict)"("DisabledEnum"=w302) -> ()  [unwired: 2 in, 2 out]
        n113 = property on="CAN Configurations" class="Arr (strict)"("DisabledEnum"=w304) -> ()  [unwired: 2 in, 2 out]
        n114 = property on="Signal to Monitor" class="Arr (strict)"("DisabledEnum"=w305) -> ()  [unwired: 2 in, 2 out]
        n115 = property on="Stop Logging" class="Bool"("DisabledEnum"=w305) -> ()  [unwired: 2 in, 2 out]
        n116 = disable-structure shown="Disabled" {
          disable-tunnel: w302 -> [w311 _]
          frame Disabled {
            n117 = property on="Preview" class="Str"("DisabledEnum"=w311) -> ()  [unwired: 2 in, 2 out]
          }
          frame Enabled {
          }
        }
        n118 = property on="Start Logging" class="Bool"("DisabledEnum"=w302) -> ()  [unwired: 2 in, 2 out]
        n119 = property on="Segment File Size" class="DigNum (strict)"("DisabledEnum"=w302) -> ()  [unwired: 2 in, 2 out]
        n120 = property on="DAQ AI Configurations" class="Arr (strict)"("DisabledEnum"=w304) -> ()  [unwired: 2 in, 2 out]
        n121 = disable-structure shown="Disabled" {
          disable-tunnel: w302 -> [w312 _]
          frame Disabled {
            n122 = property on="File size" class="DigNum (strict)"("DisabledEnum"=w312) -> ()  [unwired: 2 in, 2 out]
          }
          frame Enabled {
          }
        }
        n123 = call <vilib>:"Add State(s) to Queue__JKI_lib_State_Machine.vi"("State(s) in (\"\")"=w310) -> ("States Out"=w309:string)  [unwired: 14 in]
      }
      frame "UI: Parse Log File Name" {
        n124 = call "Parse Log File Name.vi"("Log file name"="Log file name") -> ("Parsed Log file name"=w322:string)  [unwired: 10 in]
        "Preview" <- w322
        n125 = Build Path(base path="Log file folder", name or relative path=w322) -> (appended path=w319:path)
        n126 = Bundle By Name(cluster=w324, "LogFilePath"=w319) -> (w320:T11)
        n127 = call <vilib>:"Add State(s) to Queue__JKI_lib_State_Machine.vi"("State(s) in (\"\")"=w327) -> ("States Out"=w326:string)  [unwired: 14 in]
      }
      frame "UI: CAN Update NumOfSignals" {
        n128 = local read "CAN Configurations"() -> (w330:T1[])
        n129 = for {
          tunnel: w330 -> [w337] mode=indexing
          tunnel: [w335] -> w329 mode=indexing
          n130 = Unbundle By Name(w337) -> ("XNET Cluster"=w339:refnum<k21>)
          n131 = property class="XNET Cluster"(reference=w339) -> ("Sigs"=w338:refnum<k21>[])  [unwired: 1 in, 2 out]
          n132 = Array Size(array=w338) -> (size(s)=w336:i32)
          n133 = Bundle By Name(cluster=w337, "#Signals"=w336) -> (w335:T1)
        }
        n134 = local write "CAN Configurations"(w329) -> ()
        n135 = call <vilib>:"Add State(s) to Queue__JKI_lib_State_Machine.vi"("State(s) in (\"\")"=w334) -> ("States Out"=w333:string)  [unwired: 14 in]
      }
      frame "---------- Macro ----------" {
        # "Do not put any code in this frame.\n(It is a separator no-op. You can make a copy of this frame to create a new Macro frame)"
        n136 = call <vilib>:"Add State(s) to Queue__JKI_lib_State_Machine.vi"("State(s) in (\"\")"=w344) -> ("States Out"=w343:string)  [unwired: 14 in]
      }
      frame "Macro: Initialize" {
        # "Initialization Macro\n(This is called once, when the VI starts)"
        n137 = call <vilib>:"Add State(s) to Queue__JKI_lib_State_Machine.vi"("State(s) in Front (\"\")"="Data: Initialize\nInitialize Core Data\nEvent: Register\n\nInstance Error: Obtain Error Queue\nLogger: Global Stop >> Init\n\nUI: Initialize\nUI: Front Panel State >> Open", "State(s) in (\"\")"=w350) -> ("States Out"=w349:string)  [unwired: 13 in]
      }
      frame "Macro: Start Logging" {
        n138 = Bundle By Name(cluster=w355, "Logging State"=Def-Logging_State."Logging...") -> (w353:T11)
        n139 = call <vilib>:"Add State(s) to Queue__JKI_lib_State_Machine.vi"("State(s) in Front (\"\")"="UI: Toggle Logging State\nUI: Parse Log File Name\nLogger: Data Queue: Obtain\nLogger: Global Stop >> Reset\nLogger: Writer: Launch TDMS Writer\nLogger: Readers: Launch DAQ AI Reader\nLogger: Readers: Launch XNET CAN Reader\nEvent: Control Timers >> Start\nMonitor: Initialize" ("State(s) in Front (\"\")"), "State(s) in (\"\")"=w358) -> ("States Out"=w357:string)  [unwired: 13 in]
      }
      frame "Macro: Stop Logging" {
        n140 = Bundle By Name(cluster=w363, "Logging State"=Def-Logging_State."Configuring") -> (w361:T11)
        n141 = call <vilib>:"Add State(s) to Queue__JKI_lib_State_Machine.vi"("State(s) in Front (\"\")"="UI: Toggle Logging State\nEvent: Control Timers >> Stop\nLogger: Global Stop >> Stop" ("State(s) in Front (\"\")"), "State(s) in (\"\")"=w366) -> ("States Out"=w365:string)  [unwired: 13 in]
      }
      frame "Macro: Segment File" {
        n142 = call <vilib>:"Add State(s) to Queue__JKI_lib_State_Machine.vi"("State(s) in Front (\"\")"="Logger: Global Stop >> Stop Writer\nUI: Parse Log File Name\nLogger: Writer: Launch TDMS Writer" ("State(s) in Front (\"\")"), "State(s) in (\"\")"=w372) -> ("States Out"=w371:string)  [unwired: 13 in]
      }
      frame "Macro: Exit" {
        # "Exit Macro\n(This is called once, when the VI exits)"
        n143 = Unbundle By Name(w380) -> ("Core.Close Panel on Exit?"=w379:bool)
        n144 = Select(t="UI: Front Panel State >> Close", s=w379, f="") -> (s? t:f=w376:string)
        n145 = call <vilib>:"Add State(s) to Queue__JKI_lib_State_Machine.vi"("State(s) in (\"\")"=w376, "State(s) at Back (\"\")"="Data: Cleanup\nEvent: Unregister\n\nLogger: Global Stop >> Stop\nInstance Error: Release Data Queue\n\nExit") -> ("States Out"=w374:string)  [unwired: 13 in]
        n146 = call <vilib>:"Add State(s) to Queue__JKI_lib_State_Machine.vi"("State(s) in Front (\"\")"=w374, "State(s) in (\"\")"=w383) -> ("States Out"=w382:string)  [unwired: 13 in]
      }
      frame "---------- Instance Error ----------" {
        # "Template Separator\n(You can make a copy of, or modify, this frame)"
        n147 = call <vilib>:"Add State(s) to Queue__JKI_lib_State_Machine.vi"("State(s) in (\"\")"=w388) -> ("States Out"=w387:string)  [unwired: 14 in]
      }
      frame "Instance Error: Obtain Error Queue" {
        n148 = global read "Global Variables.vi" "Const.ErrorQueueName"() -> (w394:string)
        n149 = Obtain Queue(name (unnamed)=w394, element data type=w391, error in (no error)=w391) -> (queue out=w390:refnum<queue>, error out=w393:errorcluster)  [unwired: 2 in, 1 out]
        n150 = Bundle By Name(cluster=w395, "Error Queue Ref"=w390) -> (w392:T11)
        n151 = call <vilib>:"Add State(s) to Queue__JKI_lib_State_Machine.vi"("State(s) in (\"\")"=w397) -> ("States Out"=w396:string)  [unwired: 14 in]
      }
      frame "Instance Error: Release Data Queue" {
        n152 = Unbundle By Name(w402) -> ("Error Queue Ref"=w401:refnum<queue>)
        n153 = Release Queue(queue=w401, error in (no error)=w400) -> (error out=w399:errorcluster)  [unwired: 1 in, 2 out]
        n154 = call <vilib>:"Add State(s) to Queue__JKI_lib_State_Machine.vi"("State(s) in (\"\")"=w404) -> ("States Out"=w403:string)  [unwired: 14 in]
      }
      frame "Instance Error: Handler" {
        # "Instance Error -- Display it"
        n155 = Unbundle By Name(w411) -> ("Error Queue Ref"=w410:refnum<queue>)
        n156 = Dequeue Element(queue=w410, timeout in ms (-1)=0, error in (no error)=w409) -> (element=w406:errorcluster, error out=w407:errorcluster)  [unwired: 2 out]
        n157 = call <vilib>:"General Error Handler.vi"("error in (no error)"=w406) -> ()  [unwired: 10 in, 5 out]
        n158 = call <vilib>:"Add State(s) to Queue__JKI_lib_State_Machine.vi"("State(s) in (\"\")"=w413) -> ("States Out"=w412:string)  [unwired: 14 in]
      }
      frame "---------- Logger ----------" {
        # "Template Separator\n(You can make a copy of, or modify, this frame)"
        n159 = call <vilib>:"Add State(s) to Queue__JKI_lib_State_Machine.vi"("State(s) in (\"\")"=w418) -> ("States Out"=w417:string)  [unwired: 14 in]
      }
      frame "Logger: Data Queue: Obtain" {
        n160 = global read "Global Variables.vi" "Const.TDMSDataQueueName"() -> (w425:string)
        n161 = Obtain Queue(name (unnamed)=w425, element data type=T8 {"PackageID"=0, "Data"=[]} ("Data Queue Type"), error in (no error)=w423) -> (queue out=w420:refnum<queue>, error out=w422:errorcluster)  [unwired: 2 in, 1 out]
        n162 = Bundle By Name(cluster=w426, "Data Queue Ref"=w420) -> (w421:T11)
        n163 = call <vilib>:"Add State(s) to Queue__JKI_lib_State_Machine.vi"("State(s) in (\"\")"=w428) -> ("States Out"=w427:string)  [unwired: 14 in]
      }
      frame "Logger: Data Queue: Release" {
        n164 = Unbundle By Name(w433) -> ("Data Queue Ref"=w432:T10)
        n165 = Release Queue(queue=w432, error in (no error)=w431) -> (error out=w430:errorcluster)  [unwired: 1 in, 2 out]
        n166 = call <vilib>:"Add State(s) to Queue__JKI_lib_State_Machine.vi"("State(s) in (\"\")"=w435) -> ("States Out"=w434:string)  [unwired: 14 in]
      }
      frame "Logger: Data Queue: Check State" {
        n167 = Unbundle By Name(w441) -> ("Data Queue Ref"=w440:T10)
        n168 = Get Queue Status(queue=w440, error in (no error)=w439) -> (error out=w438:errorcluster, # elements in queue=→"# elements in queue":i32)  [unwired: 1 in, 6 out]
        n169 = call <vilib>:"Add State(s) to Queue__JKI_lib_State_Machine.vi"("State(s) in (\"\")"=w443) -> ("States Out"=w442:string)  [unwired: 14 in]
      }
      frame "Logger: Writer: Launch TDMS Writer" {
        n170 = for {
          N: 50 -> [_]
          stop <- w454 stop-if-true
          n171 = global read "Global Variables.vi" "Debug.GlobalStop.WriterState"() -> (w456:bool)
          n172 = Wait (ms)(milliseconds to wait=u32 100) -> ()  [unwired: 1 out]
          n173 = Not(x=w456) -> (.not. x?=w454:bool)
        }
        n174 = Unbundle By Name(w451) -> ("LogFilePath"=w450:path)
        n175 = local read "DAQ AI Configurations"() -> (w446:T2[])
        n176 = local read "CAN Configurations"() -> (w447:T1[])
        n177 = call "Launch Action - TDMS Writer.vi"("error in (no error)"=w449, "CAN Configurations"=w447, "DAQ AI Configurations"=w446, "Log file path"=w450) -> ("error out"=w448:errorcluster)  [unwired: 7 in]
        n178 = call <vilib>:"Add State(s) to Queue__JKI_lib_State_Machine.vi"("State(s) in (\"\")"=w453) -> ("States Out"=w452:string)  [unwired: 14 in]
      }
      frame "Logger: Writer: Check File Size" {
        # "create new file to segment file"
        n179 = Unbundle By Name(w470) -> ("LogFilePath"=w469:path)
        n180 = Get File Size(file=w469, error in=w468) -> (size (in bytes)=w466:i64, 0:w467:errorcluster)  [unwired: 1 out]
        n181 = Logical Shift(y=i16 -20, x=w466) -> (x << y=w459:i64)
        "File size" <- w459
        n182 = call <vilib>:"Clear Errors.vi"("error in (no error)"=w467) -> ("error out"=w458:errorcluster)  [unwired: 5 in, 1 out]
        n183 = Greater Or Equal?(x=w459, y="Segment File Size") -> (x >= y?=w461:bool)
        n184 = Select(t="Macro: Segment File" ("State(s) at Back (\"\")"), s=w461, f="") -> (s? t:f=w457:string)
        n185 = call <vilib>:"Add State(s) to Queue__JKI_lib_State_Machine.vi"("State(s) in Front (\"\")"=w457, "State(s) in (\"\")"=w472) -> ("States Out"=w471:string)  [unwired: 13 in]
      }
      frame "Logger: Readers: Launch DAQ AI Reader" {
        n186 = call "Launch Action - DAQ AI Readers.vi"("Init PackageID"=0, "error in (no error)"=w477, "DAQ AI Configurations"="DAQ AI Configurations") -> ("error out"=w476:errorcluster)  [unwired: 8 in]
        n187 = call <vilib>:"Add State(s) to Queue__JKI_lib_State_Machine.vi"("State(s) in (\"\")"=w480) -> ("States Out"=w479:string)  [unwired: 14 in]
      }
      frame "Logger: Readers: Launch XNET CAN Reader" {
        n188 = local read "DAQ AI Configurations"() -> (w483:T2[])
        n189 = Array Size(array=w483) -> (size(s)=w482:i32)
        n190 = call "Launch Action - XNET CAN Readers.vi"("Init PackageID"=w482, "error in (no error)"=w486, "CAN Configurations"="CAN Configurations") -> ("error out"=w485:errorcluster)  [unwired: 8 in]
        n191 = call <vilib>:"Add State(s) to Queue__JKI_lib_State_Machine.vi"("State(s) in (\"\")"=w489) -> ("States Out"=w488:string)  [unwired: 14 in]
      }
      frame "Logger: Global Stop" {
        # "Template Separator\n(You can make a copy of, or modify, this frame)"
        n192 = case shown="\"Stop Writer\"" w493 {
          tunnel: w492 -> [w497 w499 w501 w504 w506]
          tunnel: [w497 w498 w500 w503 w505] -> w491
          frame Default {
          }
          frame "Init" {
            n193 = call <userlib>:"GSTOP INIT.vi"("error in (no error)"=w499) -> ("error out"=w498:errorcluster)  [unwired: 14 in]
          }
          frame "Stop", "Stop All" {
            n194 = call <userlib>:"GSTOP SET.vi"("error in (no error)"=w501) -> ("error out"=w500:errorcluster)  [unwired: 14 in]
          }
          frame "Stop Writer" {
            n195 = call <userlib>:"GSTOP SET.vi"("index(-1 for All)"=Def-GSTOP."Writer" ("GSTOP"), "error in (no error)"=w504) -> ("error out"=w503:errorcluster)  [unwired: 13 in]
          }
          frame "Reset", "Reset All" {
            (unwired) TRUE
            n196 = call <userlib>:"GSTOP RESET.vi"("error in (no error)"=w506) -> ("error out"=w505:errorcluster)  [unwired: 14 in]
          }
        }
        n197 = call <vilib>:"Add State(s) to Queue__JKI_lib_State_Machine.vi"("State(s) in (\"\")"=w496) -> ("States Out"=w495:string)  [unwired: 14 in]
      }
      frame "---------- Monitor ----------" {
        # "Template Separator\n(You can make a copy of, or modify, this frame)"
        n198 = call <vilib>:"Add State(s) to Queue__JKI_lib_State_Machine.vi"("State(s) in (\"\")"=w511) -> ("States Out"=w510:string)  [unwired: 14 in]
      }
      frame "Monitor: Initialize" {
        n199 = local read "DAQ AI Configurations"() -> (w520:T2[])
        n200 = local read "CAN Configurations"() -> (w519:T1[])
        n201 = Array Size(array=w520) -> (size(s)=w518:i32)
        n202 = Array Size(array=w519) -> (size(s)=w516:i32)
        n203 = call "Get Monitor.Names All.vi"("error in"=w526) -> ("error out"=w529:errorcluster, "Signal Names"=w517:string[])  [unwired: 9 in]
        n204 = To Variant(anything=waveform(dbl)[] [] ("Data")) -> (Variant=w523:variant)
        n205 = Compound Arithmetic op=ADD(w518, w516) -> (w513:i32)
        n206 = Initialize Array(w523, w513) -> (w522:variant[])
        n207 = Initialize Array(FALSE, w513) -> (w512:bool[])
        n208 = global write "Global Variables.vi" "Debug.GlobalStop.ReadersState"(w512) -> ()
        n209 = global write "Global Variables.vi" "Monitor.Values"(w522) -> ()
        n210 = call "Get Monitor.Units All.vi"("error in"=w529) -> ("error out"=w521:errorcluster, "Signal Units"=w525:string[])  [unwired: 9 in]
        n211 = Bundle By Name(cluster=w528, "Monitor.SignalNames"=w517, "Monitor.SignalUnits"=w525) -> (w527:T11)
        n212 = property on="Name" class="CmbBox"("Strings[]"=w517) -> ()  [unwired: 2 in, 2 out]
        n213 = call <vilib>:"Add State(s) to Queue__JKI_lib_State_Machine.vi"("State(s) in (\"\")"=w531) -> ("States Out"=w530:string)  [unwired: 14 in]
      }
      frame "Monitor: Update" {
        n214 = Unbundle By Name(w538) -> ("Monitor.SignalNames"=w537:string[])
        n215 = Unbundle By Name(w538) -> ("Monitor.SignalUnits"=w535:string[])
        n216 = call "Get Monitor.Values All.vi"("error in"=w540) -> ("error out"=w539:errorcluster, "Signal Data"=w536:waveform(dbl)[])  [unwired: 9 in]
        n217 = for {
          tunnel: w537 -> [w553]
          tunnel: w536 -> [w552]
          tunnel: w535 -> [w551]
          tunnel: "Signal to Monitor" -> [w546] mode=indexing
          tunnel: [w543] -> w533 mode=indexing
          n218 = Unbundle By Name(w546) -> ("Name"=w547:string)
          n219 = Search 1D Array(1D array=w553, element=w547) -> (index of element=w550:i32)  [unwired: 1 in]
          n220 = Index Array(array=w552, index=w550) -> (element=w549:waveform(dbl))
          n221 = Index Array(array=w551, index=w550) -> (element=w545:string)
          n222 = Unbundle By Name(w549) -> ("Y"=w548:dbl[])
          n223 = Index Array(array=w548) -> (element=w544:dbl)  [unwired: 1 in]
          n224 = Bundle By Name(cluster=w546, "Unit"=w545, "Value"=w544) -> (w543:T3)
        }
        n225 = local write "Signal to Monitor"(w533) -> ()
        n226 = call <vilib>:"Add State(s) to Queue__JKI_lib_State_Machine.vi"("State(s) in (\"\")"=w542) -> ("States Out"=w541:string)  [unwired: 14 in]
      }
    }
  }
